vi "BdcstAcquisition.vi"(8 "error in (no error)":errorcluster, 9 "Horizontal Settings":T1={"Continuous"=FALSE, "EnableAveraging"=FALSE, "Number Averages"=0, "Measurement Timeout"=0.0, "Min Record Length"=1000, "Min Sample Rate"=10000000.0, "Enforce Realtime"=TRUE, "Sampling Mode "=enum."Real Time", "Interpolation"=enum."No Interpolation", "Type"=enum."Normal", "StartTime"=0.0, "Time Per Record"=0.0, "Number of Points Minimum"=0} {"Min Sample Rate" step=1000000.0 format="%#.2p"}, 10 "ModuleID":i32) -> (0 "error out":errorcluster)   [LabVIEW 2018, in "ScopePlugins.lvlib"]
uses:
  ScopePlugins.lvlib
  ScopePluginBaseClass/Typedefs/HorizontalSettings.ctl
  ScopeShared/clEventType.ctl
  ScopeShared/ScopeShared.lvlib
  ScopePluginBaseClass/ScopePluginsBase.lvclass
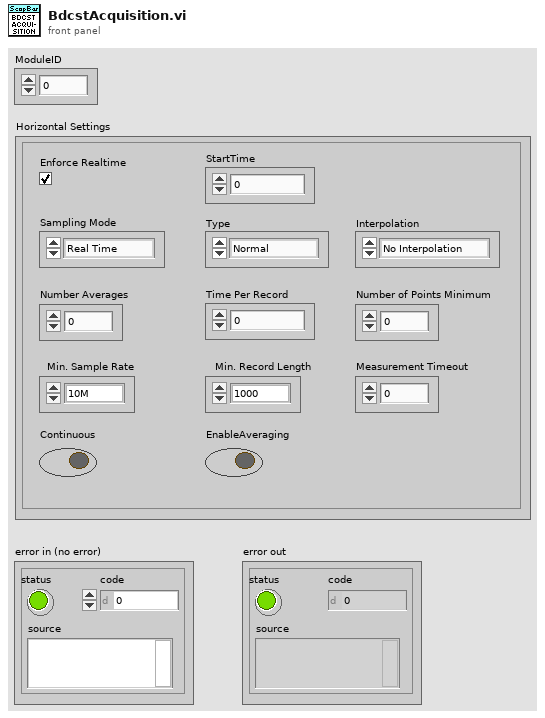
[diagram p1: front panel]
types:
  T1 = typedef "ScopePlugins.lvlib/ScopePluginsBase.lvclass/HorizontalSettings.ctl" = cluster{"Continuous":bool, "EnableAveraging":bool, "Number Averages":i32, "Measurement Timeout":dbl, "Min Record Length":i32, "Min Sample Rate":dbl, "Enforce Realtime":bool, "Sampling Mode ":enum16{"Real Time", "Equivalent Time", "Segment", "Real Time Peak Detect", "Real Time High Resolution", "Peak Detect Segment", "High Resolution Segment"}, "Interpolation":enum16{"No Interpolation", "sin(x)/x", "linear", "1 Point sin(x)/x", "2 Point sin(x)/x", "4 Point sin(x)/x", "8 Point sin(x)/x", "16 Point sin(x)/x"}, "Type":enum16{"Normal", "PeakDetect", "HighRes", "Envelope", "Average"}, "StartTime":dbl, "Time Per Record":dbl, "Number of Points Minimum":i32}
  T2 = typedef "ScopeShared.lvlib/clBroadcastEvents.ctl" = cluster{"DidInit":refnum<user-event>, "StatusUpdate":refnum<user-event>, "ErrorReport":refnum<user-event>, "DidStop":refnum<user-event>, "PathToINI":refnum<user-event>, "Handle":refnum<user-event>, "Model":refnum<user-event>, "Channels":refnum<user-event>, "Acquisition":refnum<user-event>, "Trigger":refnum<user-event>, "ExtAcquisition":refnum<user-event>, "Waveform":refnum<user-event>}
  T3 = typedef "ScopeShared.lvlib/clEventType.ctl" = cluster{"ModuleID":i32, "Data":variant}
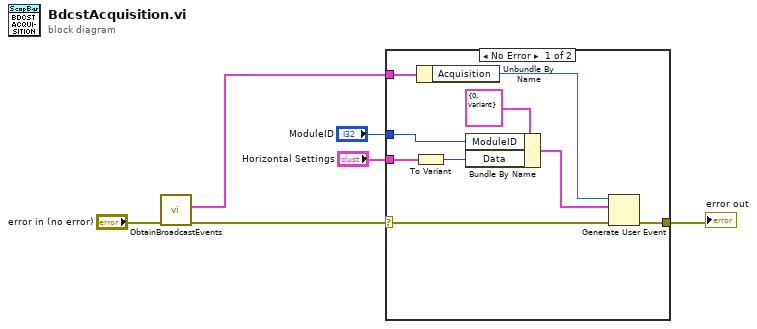
[diagram p0: block diagram]
diagram:
  n1 = call "ObtainBroadcastEvents.vi"("error in (no error)"="error in (no error)") -> ("error out"=w1:errorcluster, "clBroadcastEvents"=w6:T2)  [unwired: 9 in]
  n2 = case shown="No Error" w1 {
    selector: w1 -> [w10 w16]
    tunnel: w6 -> [w15 _]
    tunnel: "ModuleID" -> [w12 _]
    tunnel: [w8 w16] -> w4
    tunnel: "Horizontal Settings" -> [w7 _]
    frame No Error {
      n3 = To Variant(anything=w7) -> (Variant=w11:variant)
      n4 = Unbundle By Name(w15) -> ("Acquisition"=w14:refnum<user-event>)
      n5 = Bundle By Name(cluster=T3 {"ModuleID"=0, "Data"=variant} ("clEventType"), "ModuleID"=w12, "Data"=w11) -> (w9:T3)
      n6 = Generate User Event(user event=w14, event data cluster=w9, error in=w10) -> (error out=w8:errorcluster)  [unwired: 1 in, 1 out]
    }
    frame Error {
    }
  }
  "error out" <- w4
